vi "Report Error.vi"(8 "error in":errorcluster) -> (0 "error out":errorcluster)   [LabVIEW 2013, in "LVTM.lvlib"]
doc: "This VI sends error events to the main application"
uses:
  LVTM.lvlib
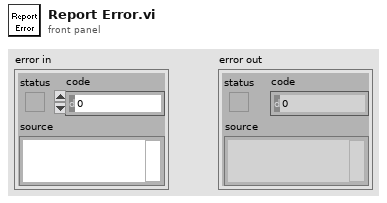
[diagram p1: front panel]
types:
  T1 = typedef "LVTM.lvlib/RequestEvents.ctl" = cluster{"Pause":refnum<user-event>, "Handle Error":refnum<user-event>, "Update Items":refnum<user-event>}
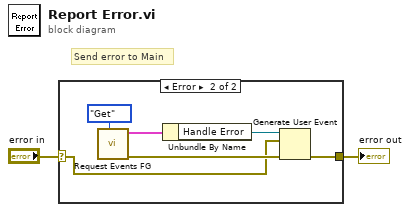
[diagram p0: block diagram]
diagram:
  # "Send error to Main"
  n1 = case shown="Error" "error in" {
    selector: "error in" -> [w3 w4]
    tunnel: [w3 w6] -> w2
    frame No Error {
    }
    frame Error {
      n2 = call "Request Events FG.vi"("Action (Get)"=enum16{"Initialize", "Get", "Destroy"}."Get" ("Action")) -> ("error out"=w5:errorcluster, "Request Events"=w8:T1)  [unwired: 9 in]
      n3 = Unbundle By Name(w8) -> ("Handle Error"=w7:refnum<user-event>)
      n4 = Generate User Event(user event=w7, event data cluster=w4, error in=w5) -> (error out=w6:errorcluster)  [unwired: 1 in, 1 out]
    }
  }
  "error out" <- w2
